vi "CRYImp wiz p3 curve layout.vi"(8 "error in (no error)":errorcluster, 9 "Data in":string[][](array[string]), 10 "Main info cluster":T2, 11 "Page flags":T1) -> (0 "error out":errorcluster, 1 "Data out":string[][](array[string]), 2 "Main info cluster out":T2, 3 "Page flags out":T1, 4 "Data array out":string[](array[string]))   [LabVIEW 2013]
uses:
  Control/CRYImp wiz page flags.ctl
  Control/CRYImp wiz main info.ctl
panel:
  in  "finish b":bool
  in  "cancel 2":bool
  out "table":string[][](table)
  out "cancel":bool
  in  "cont":bool
  in  "prev":bool
  in  "next":bool
  in  "X axis:":i32(slide) caption="aa"
  in  "Y axis:":i32(slide) caption="aa"
  in  "Data increment:":i32=1 caption="数据增加:" min=1
  in  "X axis starting row/col:":i32=1 caption="X轴开始行/列:" min=1
  in  "Y axis starting row/col:":i32=1 caption="Y轴开始行/列:" min=1
  out "X-Y data series layout":bool caption="X-Y数据系列布局"
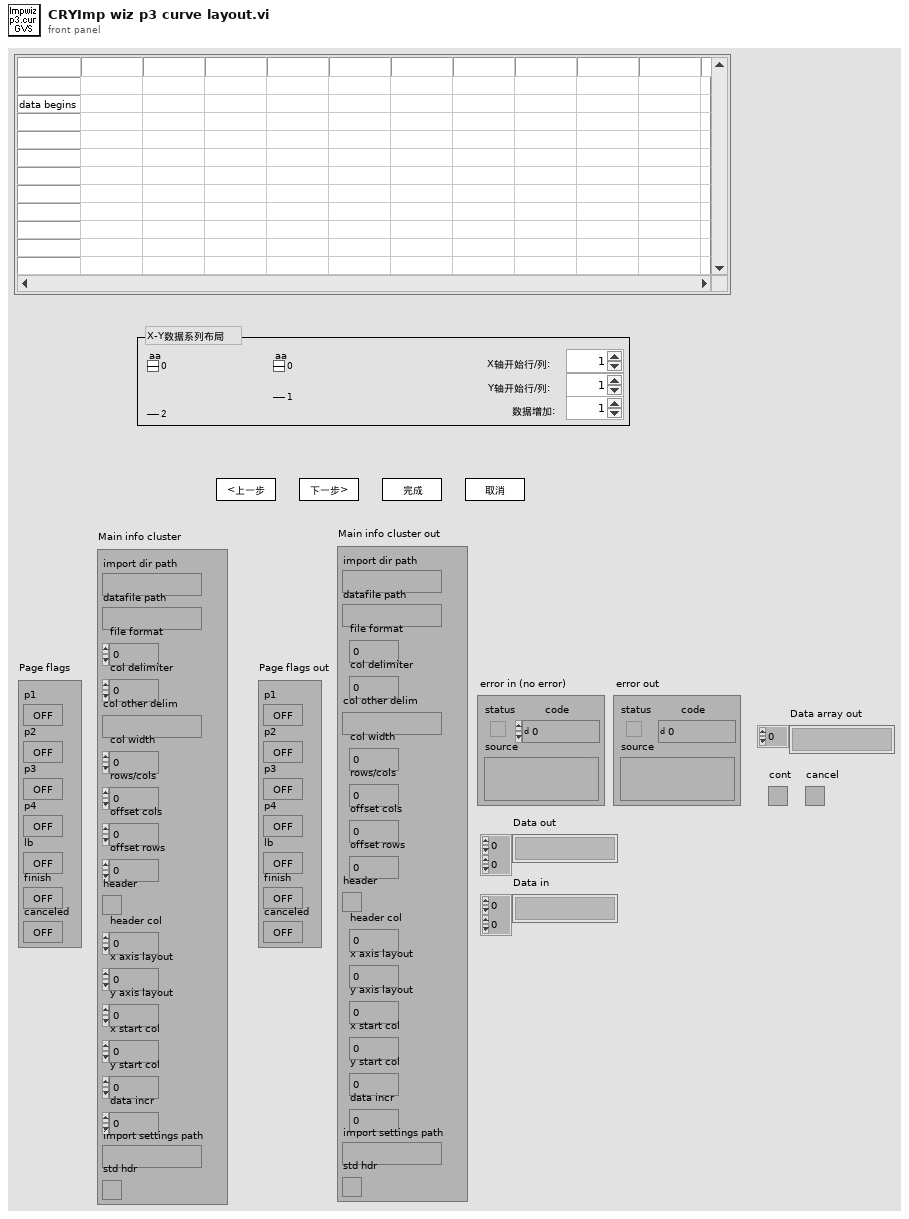
[diagram p1: front panel]
types:
  T1 = typedef "CRYImp wiz page flags.ctl" = cluster{"p1":bool, "p2":bool, "p3":bool, "p4":bool, "lb":bool, "finish":bool, "canceled":bool}
  T2 = typedef "CRYImp wiz main info.ctl" = cluster{"import dir path":path, "datafile path":path, "file format":i32, "col delimiter":i32, "col other delim":string, "col width":i32, "rows/cols":i32, "offset cols":i32, "offset rows":i32, "header":bool, "header col":i32, "x axis layout":i32, "y axis layout":i32, "x start col":i32, "y start col":i32, "data incr":i32, "import settings path":path, "std hdr":bool}
  T3 = cluster{"x col":i32, "x data type":u16, "x axis type":u16, "x prefix":string, "x unit":string, "x db ref":dbl, "y col":i32, "Name:":string, "phase incl":bool, "ym data type":u16, "ym axis type":u16, "ym prefix":string, "ym unit":string, "ym db ref":dbl, "yp data type":u16, "yp axis type":u16, "yp prefix":string, "yp unit":string, "yp db ref":dbl}
  T4 = cluster{"x col":i32, "x data type":u16, "x axis type":u16, "x prefix":string, "x unit":string, "x db ref":dbl, "y col":i32, "Name:":string, "phase incl":bool, "ym data type":u16, "ym axis type":u16, "ym prefix":string, "ym unit":string, "ym db ref":dbl, "yp data type":u16, "yp axis type":u16, "yp prefix":string, "yp unit":string, "yp db ref":dbl}[]
  T5 = cluster{"next":bool, "prev":bool, "finish b":bool, "cancel 2":bool, "X axis:":i32, "Y axis:":i32, "X axis starting row/col:":i32, "Y axis starting row/col:":i32, "Data increment:":i32, "finish":bool}
  T6 = typedef "CRYData Cluster.ctl" = cluster{"Name":string, "Curve":cluster{"x":dbl, "y":dbl, "z":dbl}[], "X data":u16, "Y data":u16, "Z data":u16, "X axis":u16, "Y axis":u16, "Z axis":u16, "X unit":string, "Y unit":string, "Z unit":string, "X dB ref":dbl, "Y dB ref":dbl, "Z dB ref":dbl, "single val":bool, "protected":bool, "display X":bool, "display Y":bool, "display Z":bool, "Test Info":string, "Step No.":i32, "Plot Settings":cluster{"Color":u32, "Interpolation":u8, "Point Style":u8, "Line Style":u8, "Point Color":u32, "Line Width":u8, "Bar Plot Style":u8, "Fill To":i16}, "AutoProtect":bool}
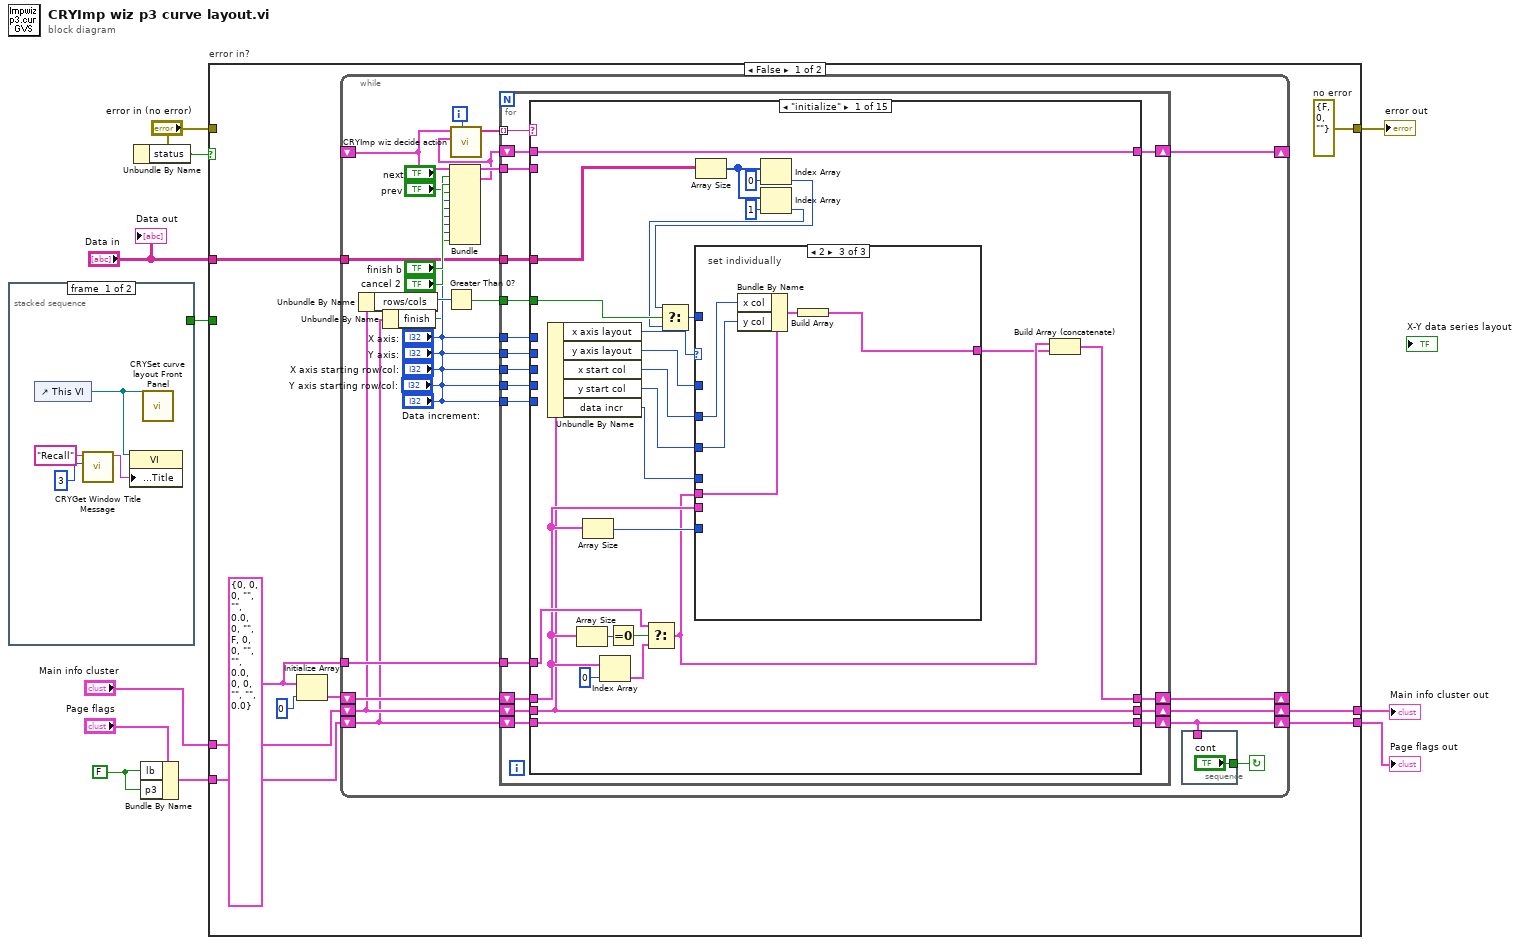
[diagram p0: block diagram]
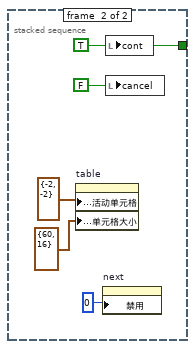
[diagram p2: hidden frame]
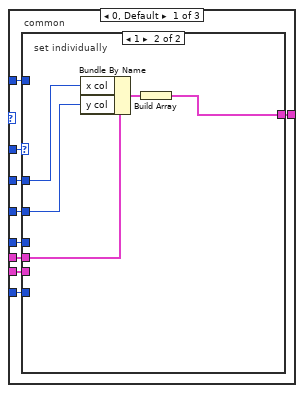
[diagram p3: hidden frame]
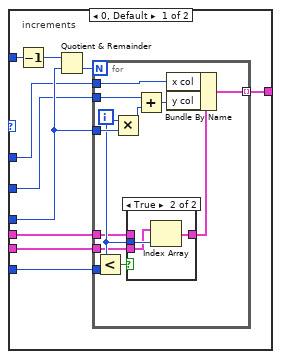
[diagram p4: hidden frame]
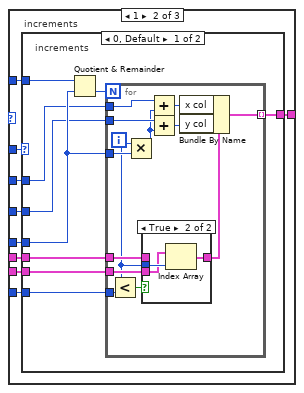
[diagram p6: hidden frame]
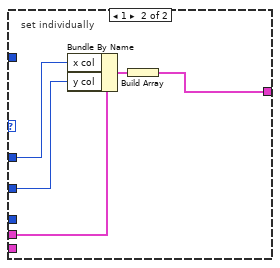
[diagram p8: hidden frame]
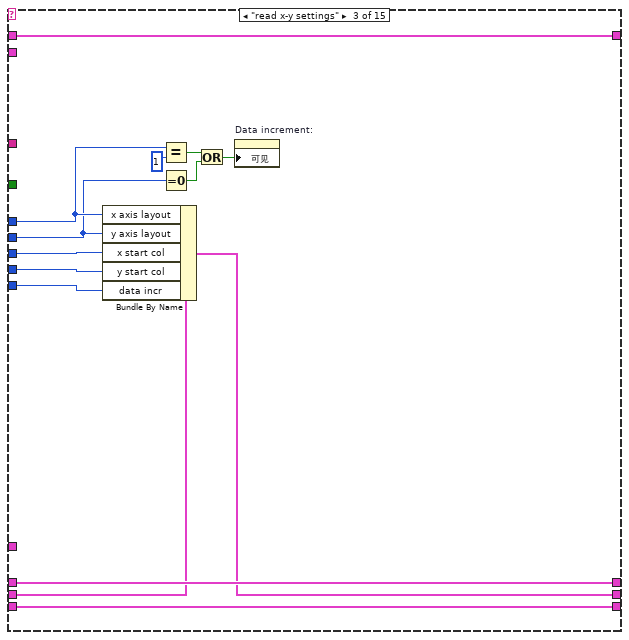
[diagram p10: hidden frame]
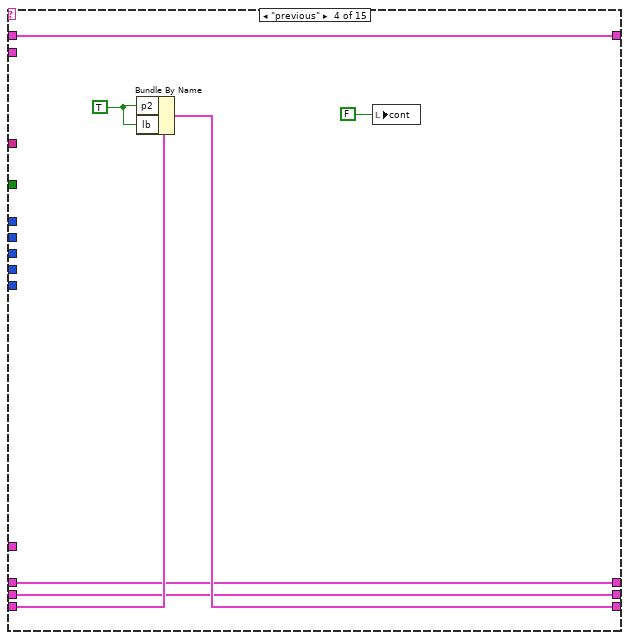
[diagram p11: hidden frame]
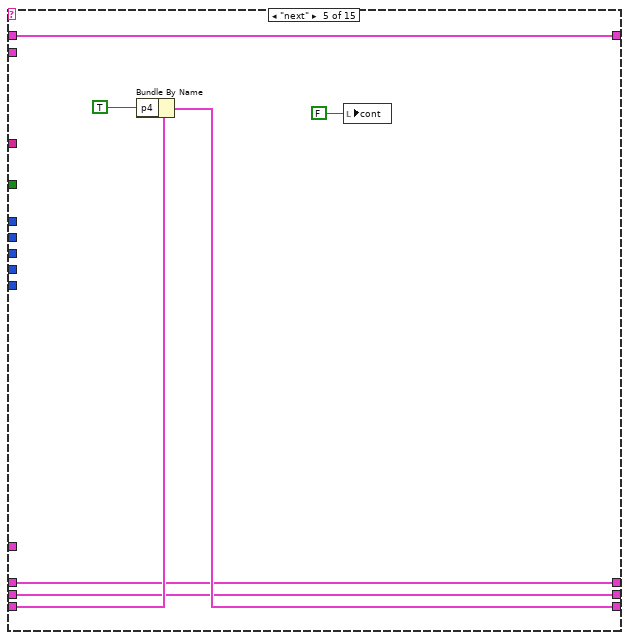
[diagram p12: hidden frame]
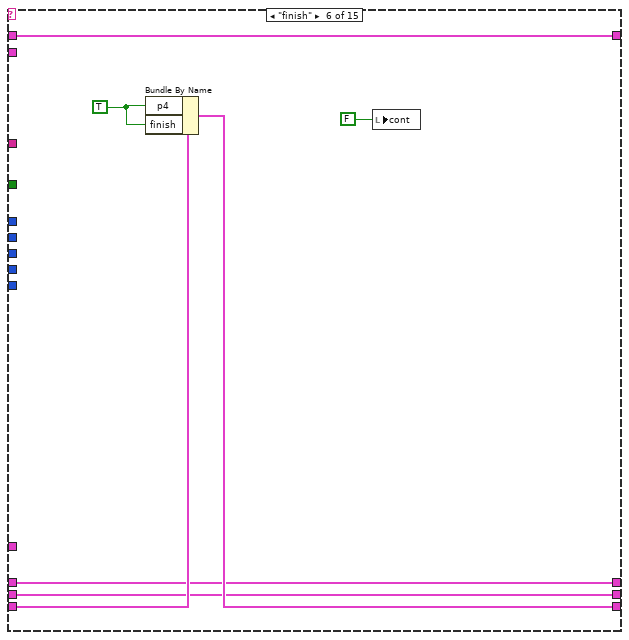
[diagram p13: hidden frame]
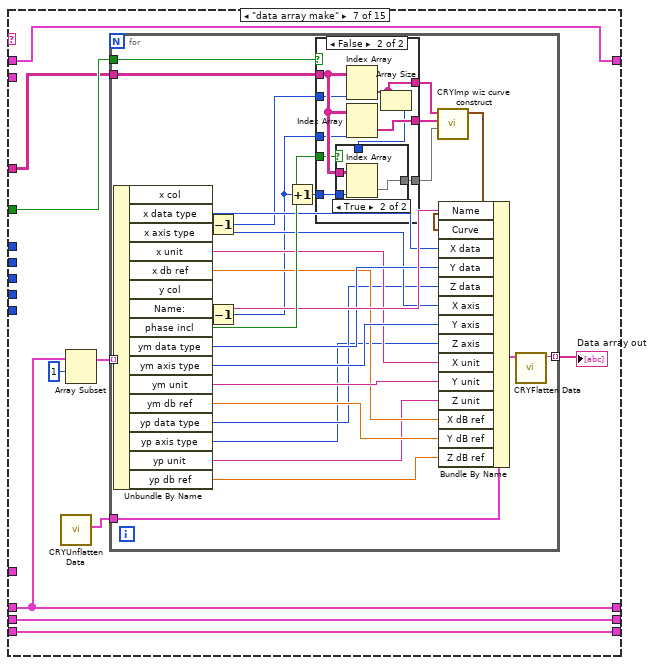
[diagram p14: hidden frame]
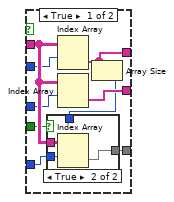
[diagram p15: hidden frame]
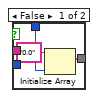
[diagram p16: hidden frame]
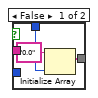
[diagram p17: hidden frame]
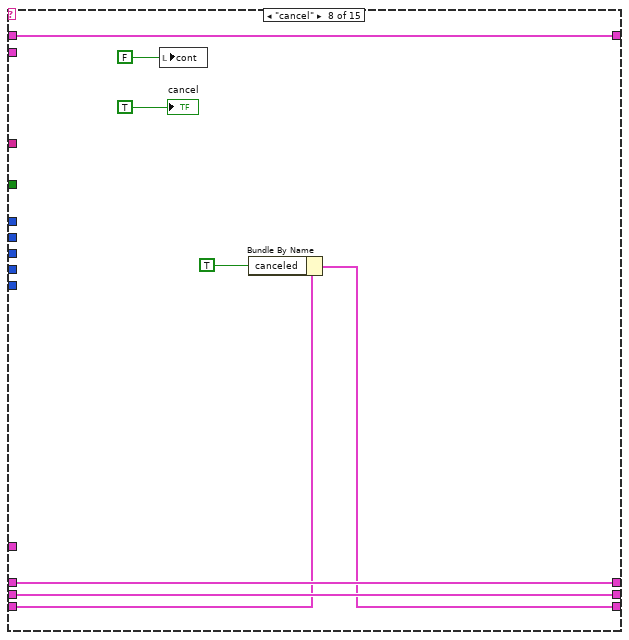
[diagram p18: hidden frame]
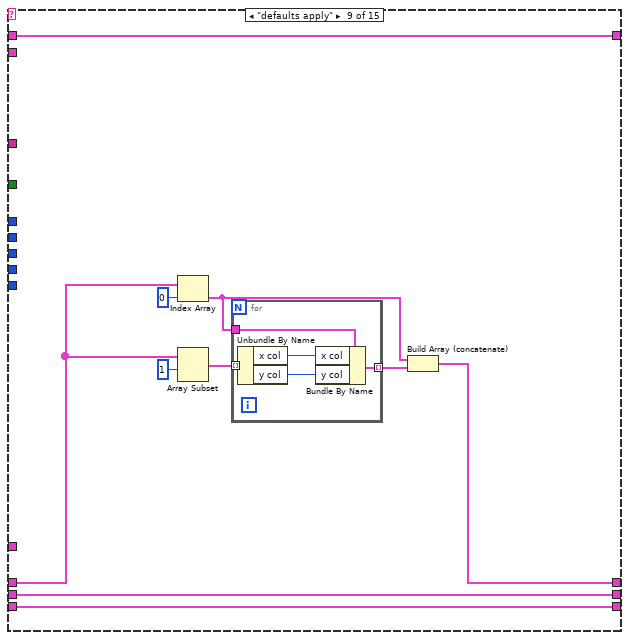
[diagram p19: hidden frame]
diagram:
  w1 = FALSE ("Bundle Element")
  n1 = stacked-sequence {
    tunnel: [_ w20] -> w11
    frame #0 {
      n2 = control-ref of="This VI"() -> (w13:refnum<vi>)
      n3 = call "CRYGet Window Title Message.vi"("No"=3, "Kind"="Recall") -> ("Multibyte String"=w12:string)  [unwired: 4 in, 5 out]
      n4 = property class="VI"(reference=w13, "Front Panel.Title"=w12) -> ()  [unwired: 1 in, 2 out]
      n5 = call "CRYSet curve layout Front Panel.vi"("Vi Ref"=w13) -> ()  [unwired: 11 in]
    }
    frame #1 {
      w20 = TRUE ("cont")
      n6 = property on="table" class="Tbl (strict)"("活动单元格:活动单元格"=cluster{i32, i32} {-2, -2} ("Write Attribute"), "活动单元格:单元格大小"=cluster{"Width":u32, "Height":u32} {"Width"=60, "Height"=16} ("Write Attribute")) -> ()  [unwired: 2 in, 2 out]
      n7 = property on="next" class="Bool"("禁用"=u8 0 ("Write Attribute")) -> ()  [unwired: 2 in, 2 out]
      n8 = local write "cont"(w20) -> ()
      n9 = local write "cancel"(FALSE ("cancelled?")) -> ()
    }
  }
  n10 = Unbundle By Name("error in (no error)") -> ("status"=w5:bool)
  n11 = Bundle By Name(cluster="Page flags", "lb"=w1, "p3"=w1) -> (w2:T1)
  n12 = case "error in?" shown="False" w5 {
    tunnel: w11 -> [_ _]
    tunnel: "Data in" -> [w27 _]
    tunnel: "Main info cluster" -> [w26 w455]
    tunnel: w2 -> [w25 w454]
    tunnel: [w24 w455] -> w8
    tunnel: [w23 w454] -> w7
    tunnel: "error in (no error)" -> [_ w456]
    tunnel: [w22 w456] -> w4
    frame False {
      w22 = errorcluster {"status"=FALSE, "code"=0, "source"=""}  # no error
      w28 = T3 {"x col"=0, "x data type"=0, "x axis type"=0, "x prefix"="", "x unit"="", "x db ref"=0.0, "y col"=0, "Name:"="", "phase incl"=FALSE, "ym data type"=0, "ym axis type"=0, "ym prefix"="", "ym unit"="", "ym db ref"=0.0, "yp data type"=0, "yp axis type"=0, "yp prefix"="", "yp unit"="", "yp db ref"=0.0} ("Output Element")
      n13 = Initialize Array(w28, 0 ("Dimension Size")) -> (w21:T4)
      n14 = while {
        shift-left: w25 -> [w31]
        shift-right: [w37] -> w23
        shift-left: w26 -> [w41]
        shift-right: [w45] -> w24
        tunnel: w28 -> [w48]
        shift-left: w21 -> [w50]
        shift-right: [w38] -> _
        shift-left: _ -> [w49]
        shift-right: [w39] -> _
        tunnel: w27 -> [w51]
        i -> [w53]
        stop <- w46 continue-if-true
        n15 = Unbundle By Name(w41) -> ("rows/cols"=w42:i32)
        n16 = Unbundle By Name(w31) -> ("finish"=w30:bool)
        n17 = Greater Than 0?(x=w42) -> (x > 0?=w47:bool)
        n18 = Bundle("next"="next", "prev"="prev", "finish b"="finish b", "cancel 2"="cancel 2", "X axis:"="X axis:", "Y axis:"="Y axis:", "X axis starting row/col:"="X axis starting row/col:", "Y axis starting row/col:"="Y axis starting row/col:", "Data increment:"="Data increment:", "finish"=w30) -> (w40:T5)  [unwired: 1 out]
        n19 = call "CRYImp wiz decide action.vi"("Iteration"=w53, "New controls"=w40, "Old controls"=w49) -> ("Frames to run"=w52:string[])  [unwired: 8 in]
        n20 = for {
          tunnel: w52 -> [w74] mode=indexing
          tunnel: w51 -> [w73]
          shift-right: [w72] -> w38
          shift-left: w50 -> [w71]
          tunnel: w47 -> [w70]
          tunnel: w49 -> [w69]
          tunnel: w48 -> [w68]
          shift-right: [w65] -> w45
          shift-left: w41 -> [w67]
          shift-right: [w64] -> w37
          shift-left: w31 -> [w66]
          shift-right: [w62] -> w39
          shift-left: w40 -> [w63]
          tunnel: "X axis:" -> [w61]
          tunnel: "Y axis:" -> [w60]
          tunnel: "X axis starting row/col:" -> [w59]
          tunnel: "Y axis starting row/col:" -> [w58]
          tunnel: "Data increment:" -> [w57]
          n21 = case shown="\"initialize\"" w74 {
            tunnel: w73 -> [w92 _ _ _ _ _ w229 _ _ _ _ _ w375 _ _]
            tunnel: [w93 w186 w201 w206 w214 w221 w232 w301 w305 w317 w321 w325 w373 w444 w453] -> w72
            tunnel: w71 -> [w84 w186 w201 w206 w214 w221 w232 w301 w309 w317 w321 w333 w373 w444 w453]
            tunnel: w70 -> [w96 _ _ _ _ _ w233 _ _ _ _ _ _ _ _]
            tunnel: w69 -> [_ _ _ _ _ _ _ _ _ _ _ w332 _ _ _]
            tunnel: w68 -> [w86 _ _ _ _ _ _ _ _ _ _ _ _ _ _]
            tunnel: w67 -> [w80 w189 w200 w207 w215 w222 w228 w298 w304 w320 w324 w340 w376 w442 w451]
            tunnel: w66 -> [w91 w188 w203 w209 w217 w224 w227 w296 w303 w319 w323 w339 w380 w443 w450]
            tunnel: [w80 w189 w199 w207 w215 w222 w228 w298 w304 w320 w324 w340 w376 w442 w451] -> w65
            tunnel: [w91 w188 w203 w208 w216 w223 w227 w295 w303 w319 w323 w339 w380 w443 w450] -> w64
            tunnel: w63 -> [w90 w187 w202 w204 w211 w218 w226 w294 w302 w318 w322 w341 w381 w445 w449]
            tunnel: [w90 w187 w202 w204 w211 w218 w226 w294 w302 w318 w322 w341 w381 w445 w449] -> w62
            tunnel: w61 -> [_ _ w195 _ _ _ _ _ _ _ _ _ _ _ _]
            tunnel: w60 -> [_ _ w193 _ _ _ _ _ _ _ _ _ _ _ _]
            tunnel: w59 -> [_ _ w198 _ _ _ _ _ _ _ _ w329 _ _ _]
            tunnel: w58 -> [_ _ w197 _ _ _ _ _ _ _ _ w328 _ _ _]
            tunnel: w57 -> [_ _ w196 _ _ _ _ _ _ _ _ _ _ _ _]
            frame "initialize" {
              n22 = Unbundle By Name(w80) -> ("x axis layout"=w75:i32, "y axis layout"=w76:i32, "x start col"=w77:i32, "y start col"=w78:i32, "data incr"=w79:i32)
              n23 = Array Size(array=w84) -> (size(s)=w88:i32)
              n24 = Array Size(array=w84) -> (size(s)=w89:i32)
              n25 = Index Array(array=w84, index=0 ("Index")) -> (element=w83:T3)
              n26 = Equal To 0?(x=w88) -> (x = 0?=w87:bool)
              n27 = Select(t=w86, s=w87, f=w83) -> (s? t:f=w82:T3)
              n28 = Array Size(array=w92) -> (size(s)=w98:i32[])
              n29 = Index Array(array=w98, index=0 ("Index")) -> (element=w95:i32)
              n30 = Index Array(array=w98, index=1 ("Index")) -> (element=w94:i32)
              n31 = Select(t=w95, s=w96, f=w94) -> (s? t:f=w97:i32)
              n32 = case shown="2" w75 {
                tunnel: w76 -> [w109 w149 _]
                tunnel: w79 -> [w108 w148 _]
                tunnel: w97 -> [w107 w147 _]
                tunnel: w82 -> [w106 w146 w184]
                tunnel: [w105 w145 w183] -> w81
                tunnel: w77 -> [w104 w144 w182]
                tunnel: w78 -> [w103 w143 w181]
                tunnel: w84 -> [w102 w142 _]
                tunnel: w89 -> [w101 w141 _]
                frame 0, Default {
                  # "common"
                  n33 = case shown="1" w109 {
                    tunnel: w108 -> [w114 _]
                    tunnel: w107 -> [w119 _]
                    tunnel: w106 -> [w116 w140]
                    tunnel: [w115 w138] -> w105
                    tunnel: w104 -> [w113 w137]
                    tunnel: w103 -> [w112 w136]
                    tunnel: w102 -> [w111 _]
                    tunnel: w101 -> [w110 _]
                    frame 0, Default {
                      # "increments"
                      n34 = Decrement(x=w119) -> (x-1=w118:i32)
                      n35 = Quotient & Remainder(x=w118, y=w114) -> (floor(x/y)=w117:i32)  [unwired: 1 out]
                      n36 = for {
                        N: w117 -> [_]
                        tunnel: w116 -> [w121]
                        tunnel: [w130] -> w115 mode=indexing
                        tunnel: w114 -> [w129]
                        tunnel: w113 -> [w127]
                        tunnel: w112 -> [w126]
                        tunnel: w111 -> [w122]
                        tunnel: w110 -> [w125]
                        i -> [w123]
                        n37 = Less?(x=w123, y=w125) -> (x < y?=w124:bool)
                        n38 = Multiply(x=w123, y=w129) -> (x*y=w128:i32)
                        n39 = case shown="True" w124 {
                          tunnel: w123 -> [_ w135]
                          tunnel: w122 -> [_ w134]
                          tunnel: w121 -> [w132 _]
                          tunnel: [w132 w133] -> w120
                          frame False {
                          }
                          frame True {
                            n40 = Index Array(array=w134, index=w135) -> (element=w133:T3)
                          }
                        }
                        n41 = Add(x=w126, y=w128) -> (x+y=w131:i32)
                        n42 = Bundle By Name(cluster=w120, "x col"=w127, "y col"=w131) -> (w130:T3)
                      }
                    }
                    frame 1 {
                      # "set individually"
                      n43 = Bundle By Name(cluster=w140, "x col"=w137, "y col"=w136) -> (w139:T3)
                      n44 = Build Array(w139) -> (w138:T4)
                    }
                  }
                }
                frame 1 {
                  # "increments"
                  n45 = case shown="0, Default" w149 {
                    tunnel: w148 -> [w155 _]
                    tunnel: w147 -> [w152 _]
                    tunnel: w146 -> [w157 w180]
                    tunnel: [w156 w178] -> w145
                    tunnel: w144 -> [w154 w177]
                    tunnel: w143 -> [w153 w176]
                    tunnel: w142 -> [w151 _]
                    tunnel: w141 -> [w150 _]
                    frame 0, Default {
                      # "increments"
                      n46 = Quotient & Remainder(x=w152, y=w155) -> (floor(x/y)=w158:i32)  [unwired: 1 out]
                      n47 = for {
                        N: w158 -> [_]
                        tunnel: w157 -> [w163]
                        tunnel: [w170] -> w156 mode=indexing
                        tunnel: w155 -> [w169]
                        tunnel: w154 -> [w167]
                        tunnel: w153 -> [w168]
                        tunnel: w151 -> [w162]
                        tunnel: w150 -> [w161]
                        i -> [w160]
                        n48 = Less?(x=w160, y=w161) -> (x < y?=w164:bool)
                        n49 = Multiply(x=w160, y=w169) -> (x*y=w166:i32)
                        n50 = case shown="True" w164 {
                          tunnel: w160 -> [_ w175]
                          tunnel: w162 -> [_ w174]
                          tunnel: w163 -> [w172 _]
                          tunnel: [w172 w173] -> w159
                          frame False {
                          }
                          frame True {
                            n51 = Index Array(array=w174, index=w175) -> (element=w173:T3)
                          }
                        }
                        n52 = Add(x=w167, y=w166) -> (x+y=w165:i32)
                        n53 = Add(x=w168, y=w166) -> (x+y=w171:i32)
                        n54 = Bundle By Name(cluster=w159, "x col"=w165, "y col"=w171) -> (w170:T3)
                      }
                    }
                    frame 1 {
                      # "set individually"
                      n55 = Bundle By Name(cluster=w180, "x col"=w177, "y col"=w176) -> (w179:T3)
                      n56 = Build Array(w179) -> (w178:T4)
                    }
                  }
                }
                frame 2 {
                  # "set individually"
                  n57 = Bundle By Name(cluster=w184, "x col"=w182, "y col"=w181) -> (w185:T3)
                  n58 = Build Array(w185) -> (w183:T4)
                }
              }
              n59 = Build Array (concatenate)(w82, w81) -> (w93:T4)
            }
            frame "update x-y settings" {
            }
            frame "read x-y settings" {
              n60 = Bundle By Name(cluster=w200, "x axis layout"=w195, "y axis layout"=w193, "x start col"=w198, "y start col"=w197, "data incr"=w196) -> (w199:T2)
              n61 = Equal?(x=w195, y=1) -> (x = y?=w192:bool)
              n62 = Equal To 0?(x=w193) -> (x = 0?=w191:bool)
              n63 = Or(x=w192, y=w191) -> (x .or. y?=w190:bool)
              n64 = property on="Data increment:" class="DigNum (strict)"("可见"=w190) -> ()  [unwired: 2 in, 2 out]
            }
            frame "previous" {
              w210 = TRUE ("Bundle Element")
              n65 = Bundle By Name(cluster=w209, "p2"=w210, "lb"=w210) -> (w208:T1)
              n66 = local write "cont"(FALSE ("cont")) -> ()
            }
            frame "next" {
              n67 = Bundle By Name(cluster=w217, "p4"=TRUE ("Bundle Element")) -> (w216:T1)
              n68 = local write "cont"(FALSE ("cont")) -> ()
            }
            frame "finish" {
              w220 = TRUE ("Bundle Element")
              n69 = Bundle By Name(cluster=w224, "p4"=w220, "finish"=w220) -> (w223:T1)
              n70 = local write "cont"(FALSE ("cont")) -> ()
            }
            frame "data array make" {
              n71 = call "CRYUnflatten Data.vi"() -> ("Datum"=w234:T6)  [unwired: 9 in, 2 out]
              n72 = Array Subset(array=w232, index=1 ("Array Index")) -> (w231:T4)  [unwired: 1 in]
              n73 = for {
                tunnel: w231 -> [w263] mode=indexing
                tunnel: w234 -> [w262]
                tunnel: w233 -> [w261]
                tunnel: w229 -> [w260]
                tunnel: [w241] -> w225 mode=indexing
                n74 = Unbundle By Name(w263) -> ("x col"=w257:i32, "x data type"=w254:u16, "x axis type"=w252:u16, "x unit"=w250:string, "x db ref"=w248:dbl, "y col"=w256:i32, "Name:"=w258:string, "phase incl"=w259:bool, "ym data type"=w253:u16, "ym axis type"=w251:u16, "ym unit"=w249:string, "ym db ref"=w247:dbl, "yp data type"=w246:u16, "yp axis type"=w245:u16, "yp unit"=w244:string, "yp db ref"=w243:dbl)
                n75 = Decrement(x=w257) -> (x-1=w240:i32)
                n76 = Decrement(x=w256) -> (x-1=w239:i32)
                n77 = Increment(x=w239) -> (x+1=w255:i32)
                n78 = case shown="False" w261 {
                  tunnel: w260 -> [w272 w287]
                  tunnel: w259 -> [w271 w286]
                  tunnel: w240 -> [w270 w281]
                  tunnel: w239 -> [w269 w280]
                  tunnel: w255 -> [w268 w279]
                  tunnel: [w265 w283] -> w237
                  tunnel: [w267 w285] -> w238
                  tunnel: [w266 w284] -> w236
                  frame True {
                    n79 = Index Array(array=w272, index (row)=w270) -> (element=w265:string[])  [unwired: 1 in]
                    n80 = Index Array(array=w272, index (row)=w269) -> (element=w267:string[])  [unwired: 1 in]
                    n81 = Array Size(array=w265) -> (size(s)=w264:i32)
                    n82 = case shown="True" w271 {
                      tunnel: w272 -> [_ w278]
                      tunnel: w268 -> [_ w277]
                      tunnel: [w273 w276] -> w266
                      tunnel: w264 -> [w275 _]
                      frame False {
                        n83 = Initialize Array("0.0", w275) -> (w273:string[])
                      }
                      frame True {
                        n84 = Index Array(array=w278, index (row)=w277) -> (element=w276:string[])  [unwired: 1 in]
                      }
                    }
                  }
                  frame False {
                    n85 = Index Array(array=w287, index (col)=w281) -> (element=w283:string[])  [unwired: 1 in]
                    n86 = Index Array(array=w287, index (col)=w280) -> (element=w285:string[])  [unwired: 1 in]
                    n87 = Array Size(array=w283) -> (size(s)=w282:i32)
                    n88 = case shown="True" w286 {
                      tunnel: w287 -> [_ w293]
                      tunnel: [w288 w292] -> w284
                      tunnel: w282 -> [w290 _]
                      tunnel: w279 -> [_ w291]
                      frame False {
                        n89 = Initialize Array("0.0", w290) -> (w288:string[])
                      }
                      frame True {
                        n90 = Index Array(array=w293, index (col)=w291) -> (element=w292:string[])  [unwired: 1 in]
                      }
                    }
                  }
                }
                n91 = call "CRYImp wiz curve construct.vi"("Z strings"=w236, "Y strings"=w238, "X strings"=w237) -> ("Curve"=w235:cluster{"x":dbl, "y":dbl, "z":dbl}[])  [unwired: 8 in]
                n92 = Bundle By Name(cluster=w262, "Name"=w258, "Curve"=w235, "X data"=w254, "Y data"=w253, "Z data"=w246, "X axis"=w252, "Y axis"=w251, "Z axis"=w245, "X unit"=w250, "Y unit"=w249, "Z unit"=w244, "X dB ref"=w248, "Y dB ref"=w247, "Z dB ref"=w243) -> (w242:T6)
                n93 = call "CRYFlatten Data.vi"("Datum"=w242) -> ("Data flattened"=w241:string)  [unwired: 10 in]
              }
              "Data array out" <- w225
            }
            frame "cancel" {
              n94 = local write "cont"(FALSE ("cont")) -> ()
              n95 = Bundle By Name(cluster=w296, "canceled"=TRUE ("Bundle Element")) -> (w295:T1)
              "cancel" <- TRUE ("cancelled?")
            }
            frame "defaults apply" {
              n96 = Index Array(array=w309, index=0 ("Index")) -> (element=w306:T3)
              n97 = Array Subset(array=w309, index=1 ("Array Index")) -> (w308:T4)  [unwired: 1 in]
              n98 = for {
                tunnel: w308 -> [w316] mode=indexing
                tunnel: w306 -> [w315]
                tunnel: [w312] -> w307 mode=indexing
                n99 = Unbundle By Name(w316) -> ("x col"=w314:i32, "y col"=w313:i32)
                n100 = Bundle By Name(cluster=w315, "x col"=w314, "y col"=w313) -> (w312:T3)
              }
              n101 = Build Array (concatenate)(w306, w307) -> (w305:T4)
            }
            frame "add series" {
            }
            frame "remove series" {
            }
            frame "col shift" {
              n102 = Unbundle By Name(w332) -> ("X axis starting row/col:"=w331:i32, "Y axis starting row/col:"=w330:i32)
              n103 = Subtract(x=w329, y=w331) -> (x-y=w327:i32)
              n104 = Subtract(x=w328, y=w330) -> (x-y=w326:i32)
              n105 = Index Array(array=w333, index=0 ("Index")) -> (element=w334:T3)
              n106 = Array Subset(array=w333, index=1 ("Array Index")) -> (w336:T4)  [unwired: 1 in]
              n107 = for {
                tunnel: w336 -> [w344] mode=indexing
                tunnel: [w349] -> w335 mode=indexing
                tunnel: w327 -> [w343]
                tunnel: w326 -> [w342]
                n108 = Unbundle By Name(w344) -> ("x col"=w348:i32, "y col"=w347:i32)
                n109 = Add(x=w348, y=w343) -> (x+y=w346:i32)
                n110 = Add(x=w347, y=w342) -> (x+y=w345:i32)
                n111 = Bundle By Name(cluster=w344, "x col"=w346, "y col"=w345) -> (w349:T3)
              }
              n112 = Build Array (concatenate)(w334, w335) -> (w325:T4)
            }
            frame "table update" {
              w354 = ""
              w359 = 0 ("Index")
              w350 = FALSE  # (no need for header indicator here)
              n113 = Array Size(array=w375) -> (size(s)=w377:i32[])
              n114 = Unbundle By Name(w376) -> ("rows/cols"=w361:i32, "header col"=w360:i32, "x axis layout"=w352:i32)  [unwired: 1 out]
              n115 = for {
                tunnel: w373 -> [w417] mode=indexing
                tunnel: [w414] -> w362 mode=indexing
                n116 = Unbundle By Name(w417) -> ("x col"=w416:i32, "y col"=w415:i32)
                n117 = Bundle("x col"=w416, "y col"=w415) -> (w414:cluster{"x col":i32, "y col":i32})  [unwired: 1 out]
              }
              n118 = Index Array(array=w377, index=0 ("Index")) -> (element=w358:i32)
              n119 = Index Array(array=w377, index=1 ("Index")) -> (element=w357:i32)
              n120 = Decrement(x=w360) -> (x-1=w353:i32)
              n121 = Equal To 0?(x=w352) -> (x = 0?=w351:bool)
              n122 = case shown="0, Default" w361 {
                tunnel: w357 -> [w425 _]
                tunnel: w375 -> [w423 w433]
                tunnel: w358 -> [_ w434]
                tunnel: [w422 w430] -> w374
                tunnel: w362 -> [w419 w427]
                tunnel: w351 -> [w418 w426]
                frame 0, Default {
                  n123 = Initialize Array("", w425) -> (w421:string[])
                  n124 = call "CRYHeader x-y cols assign.vi"("Common x-axis"=w418, "Column assignments"=w419, "Header row, empty"=w421) -> ("Header row out"=w420:string[])  [unwired: 8 in]
                  n125 = Build Array (concatenate)(w420, w423) -> (w422:string[][])
                }
                frame 1 {
                  n126 = Transpose 2D Array(2D array=w433) -> (transposed array=w432:string[][])
                  n127 = Initialize Array("", w434) -> (w429:string[])
                  n128 = call "CRYHeader x-y cols assign.vi"("Common x-axis"=w426, "Column assignments"=w427, "Header row, empty"=w429) -> ("Header row out"=w428:string[])  [unwired: 8 in]
                  n129 = Build Array (concatenate)(w428, w432) -> (w431:string[][])
                  n130 = Transpose 2D Array(2D array=w431) -> (transposed array=w430:string[][])
                }
              }
              "table" <- w374
              n131 = Subtract(x=w358, y=w359) -> (x-y=w365:i32)
              n132 = Subtract(x=w357, y=w359) -> (x-y=w364:i32)
              n133 = for {
                N: w365 -> [_]
                tunnel: "row %d" -> [w411]
                tunnel: [w410] -> w367 mode=indexing
                i -> [w413]
                n134 = Increment(x=w413) -> (x+1=w412:i32)
                n135 = Format Into String(format string=w411, w412) -> (resulting string=w410:string)  [unwired: 2 in, 1 out]
              }
              n136 = for {
                N: w364 -> [_]
                tunnel: "col %d" -> [w407]
                tunnel: [w406] -> w369 mode=indexing
                i -> [w409]
                n137 = Increment(x=w409) -> (x+1=w408:i32)
                n138 = Format Into String(format string=w407, w408) -> (resulting string=w406:string)  [unwired: 2 in, 1 out]
              }
              n139 = Initialize Array(w354, w359) -> (w370:string[])
              n140 = Initialize Array(w354, w359) -> (w368:string[])
              n141 = case shown="1" w361 {
                tunnel: [w389 w394] -> w355
                tunnel: [w382 w403] -> w356
                tunnel: w370 -> [w393 w405]
                tunnel: w369 -> [w392 _]
                tunnel: w368 -> [w391 w404]
                tunnel: w367 -> [_ w402]
                tunnel: "data begins" -> [w390 w401]
                tunnel: "header" -> [w387 w399]
                tunnel: w350 -> [w386 w398]
                tunnel: w353 -> [w385 w397]
                tunnel: w354 -> [w384 w396]
                frame 0, Default {
                  n142 = Build Array (concatenate)(w391, w390) -> (w388:string[])
                  n143 = Build Array (concatenate)(w393, w392) -> (w389:string[])
                  n144 = call "CRYArray replace with extend.vi"("Enable (T)"=w386, "Index"=w385, "String element"=w387, "String array"=w388) -> ("String array out"=w383:string[])  [unwired: 7 in]
                  n145 = Build Array (concatenate)(w384, w383) -> (w382:string[])
                }
                frame 1 {
                  n146 = Build Array (concatenate)(w404, w402) -> (w403:string[])
                  n147 = Build Array (concatenate)(w405, w401) -> (w400:string[])
                  n148 = call "CRYArray replace with extend.vi"("Enable (T)"=w398, "Index"=w397, "String element"=w399, "String array"=w400) -> ("String array out"=w395:string[])  [unwired: 7 in]
                  n149 = Build Array (concatenate)(w396, w395) -> (w394:string[])
                }
              }
              n150 = property on="table" class="Tbl (strict)"("行首字符串[]"=w356, "列首字符串[]"=w355) -> ()  [unwired: 2 in, 2 out]
            }
            frame "init settings" {
              n151 = Unbundle By Name(w442) -> ("x axis layout"=w437:i32, "y axis layout"=w436:i32, "x start col"=w448:i32, "y start col"=w447:i32, "data incr"=w446:i32)
              n152 = local write "X axis starting row/col:"(w448) -> ()
              n153 = local write "Y axis starting row/col:"(w447) -> ()
              n154 = local write "Data increment:"(w446) -> ()
              n155 = local write "X axis:"(w437) -> ()
              n156 = local write "Y axis:"(w436) -> ()
              n157 = Equal?(x=w437, y=1) -> (x = y?=w440:bool)
              n158 = Equal To 0?(x=w436) -> (x = 0?=w439:bool)
              n159 = Or(x=w440, y=w439) -> (x .or. y?=w438:bool)
              n160 = property on="Data increment:" class="DigNum (strict)"("可见"=w438) -> ()  [unwired: 2 in, 2 out]
            }
            frame "idle", Default {
              n161 = Wait (ms)(milliseconds to wait=u32 150) -> ()  [unwired: 1 out]
            }
          }
        }
        n162 = stacked-sequence {
          tunnel: ["cont"] -> w46
          tunnel: w37 -> [_]
          frame #0 {
          }
        }
      }
    }
    frame True {
    }
  }
  "Page flags out" <- w7
  "Main info cluster out" <- w8
  "error out" <- w4
  "Data out" <- "Data in"
